vi "0516205_鍾禾翊_HW1.vi"() -> ()   [LabVIEW 2018]
panel:
  out "Boolean 28":bool
  out "Boolean 27":bool
  out "Boolean 26":bool
  out "Boolean 25":bool
  out "Boolean 24":bool
  out "Boolean 23":bool
  out "Boolean 22":bool
  out "Boolean 21":bool
  out "Boolean 20":bool
  out "Boolean 19":bool
  out "Boolean 18":bool
  out "Boolean 17":bool
  out "Boolean 16":bool
  out "Boolean 15":bool
  in  "Tank 2":i32
  out "Boolean 14":bool
  out "Boolean 13":bool
  out "Boolean 12":bool
  out "Boolean 11":bool
  out "Boolean 10":bool
  out "Boolean 9":bool
  out "Boolean 8":bool
  in  "stop":bool
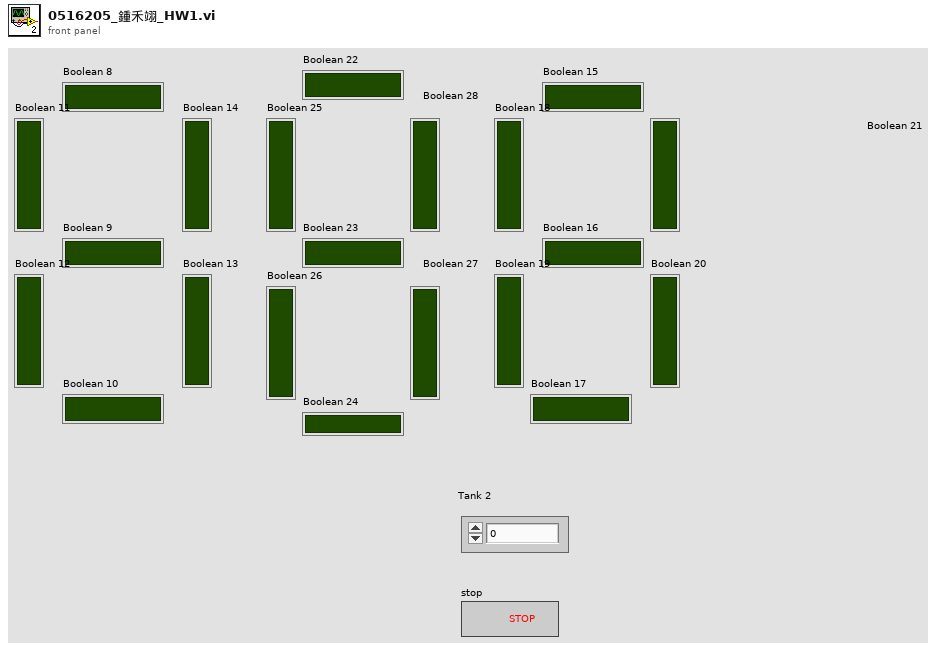
[diagram p1: front panel]
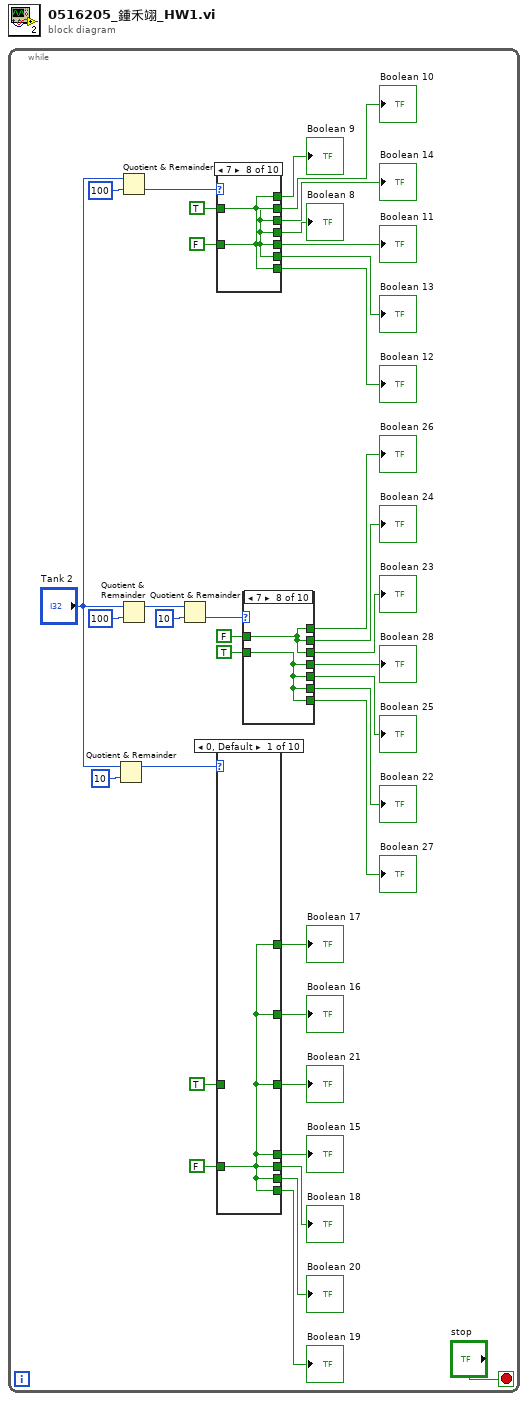
[diagram p0: block diagram]
diagram:
  n1 = while {
    stop <- "stop" stop-if-true
    n2 = Quotient & Remainder(x="Tank 2", y=10) -> (x-y*floor(x/y)=w1:i32)  [unwired: 1 out]
    n3 = Quotient & Remainder(x="Tank 2", y=100) -> (floor(x/y)=w7:i32)  [unwired: 1 out]
    n4 = Quotient & Remainder(x="Tank 2", y=100) -> (x-y*floor(x/y)=w6:i32)  [unwired: 1 out]
    n5 = Quotient & Remainder(x=w6, y=10) -> (floor(x/y)=w4:i32)  [unwired: 1 out]
    n6 = case shown="7" w7 {
      tunnel: [w74 w75 w77 w79 w82 w83 w85 w87 w89 w90] -> w36
      tunnel: [w74 w75 w78 w80 w81 w83 w85 w87 w89 w90] -> w30
      tunnel: [w74 w76 w77 w79 w81 w84 w86 w87 w89 w90] -> w35
      tunnel: [w74 w75 w77 w79 w81 w83 w85 w88 w89 w90] -> w34
      tunnel: [w74 w75 w78 w79 w82 w84 w85 w88 w89 w91] -> w33
      tunnel: [w74 w76 w77 w80 w81 w83 w85 w87 w89 w90] -> w32
      tunnel: [w74 w75 w77 w79 w82 w83 w85 w88 w89 w90] -> w31
      tunnel: TRUE -> [_ w76 w77 w79 w81 w83 w85 w87 w89 w90]
      tunnel: FALSE -> [w74 w75 w78 w80 w82 w84 w86 w88 _ w91]
      frame 0, Default {
      }
      frame 1 {
      }
      frame 3 {
      }
      frame 2 {
      }
      frame 4 {
      }
      frame 5 {
      }
      frame 6 {
      }
      frame 7 {
      }
      frame 8 {
      }
      frame 9 {
      }
    }
    "Boolean 8" <- w36
    "Boolean 9" <- w34
    "Boolean 10" <- w31
    "Boolean 11" <- w30
    "Boolean 12" <- w33
    "Boolean 13" <- w32
    "Boolean 14" <- w35
    n7 = case shown="0, Default" w1 {
      tunnel: [w56 w57 w59 w61 w64 w65 w67 w69 w71 w72] -> w26
      tunnel: [w56 w57 w60 w62 w63 w65 w67 w69 w71 w72] -> w20
      tunnel: [w56 w58 w59 w61 w63 w66 w68 w69 w71 w72] -> w25
      tunnel: [w56 w57 w59 w61 w63 w65 w67 w70 w71 w72] -> w24
      tunnel: [w56 w57 w60 w61 w64 w66 w67 w70 w71 w73] -> w23
      tunnel: [w56 w58 w59 w62 w63 w65 w67 w69 w71 w72] -> w22
      tunnel: [w56 w57 w59 w61 w64 w65 w67 w70 w71 w72] -> w21
      tunnel: TRUE -> [_ w58 w59 w61 w63 w65 w67 w69 w71 w72]
      tunnel: FALSE -> [w56 w57 w60 w62 w64 w66 w68 w70 _ w73]
      frame 0, Default {
      }
      frame 1 {
      }
      frame 3 {
      }
      frame 2 {
      }
      frame 4 {
      }
      frame 5 {
      }
      frame 6 {
      }
      frame 7 {
      }
      frame 8 {
      }
      frame 9 {
      }
    }
    "Boolean 15" <- w26
    "Boolean 16" <- w24
    "Boolean 17" <- w21
    "Boolean 18" <- w20
    "Boolean 19" <- w23
    "Boolean 20" <- w22
    "Boolean 21" <- w25
    n8 = case shown="7" w4 {
      tunnel: [w38 w39 w41 w43 w46 w47 w49 w51 w53 w54] -> w17
      tunnel: [w38 w39 w42 w44 w45 w47 w49 w51 w53 w54] -> w11
      tunnel: [w38 w40 w41 w43 w45 w48 w50 w51 w53 w54] -> w16
      tunnel: [w38 w39 w41 w43 w45 w47 w49 w52 w53 w54] -> w15
      tunnel: [w38 w39 w42 w43 w46 w48 w49 w52 w53 w55] -> w14
      tunnel: [w38 w40 w41 w44 w45 w47 w49 w51 w53 w54] -> w13
      tunnel: [w38 w39 w41 w43 w46 w47 w49 w52 w53 w54] -> w12
      tunnel: TRUE -> [_ w40 w41 w43 w45 w47 w49 w51 w53 w54]
      tunnel: FALSE -> [w38 w39 w42 w44 w46 w48 w50 w52 _ w55]
      frame 0, Default {
      }
      frame 1 {
      }
      frame 3 {
      }
      frame 2 {
      }
      frame 4 {
      }
      frame 5 {
      }
      frame 6 {
      }
      frame 7 {
      }
      frame 8 {
      }
      frame 9 {
      }
    }
    "Boolean 22" <- w17
    "Boolean 23" <- w15
    "Boolean 24" <- w12
    "Boolean 25" <- w11
    "Boolean 26" <- w14
    "Boolean 27" <- w13
    "Boolean 28" <- w16
  }
